vi "GetMicronArgs.vi"(8 "error in (no error)":errorcluster, 10 "Args":string[](array[string]), 11 "Default Connection String":string="localhost:50051") -> (0 "error out":errorcluster, 3 "Micron Args":T1)   [LabVIEW 2019, in "MicronServer.lvlib" / "ServiceBase.lvclass"]
uses:
  ServiceBase.lvclass
  Typedefs/MicronArgs.ctl
  <vilib>/Wiresmith Technology/G CLI/Argument Parser/Option Class/Option Configuration.ctl
  <vilib>/Wiresmith Technology/G CLI/Argument Parser/Option Class/Argument Type.ctl
  <vilib>/SLL Toolkit/SLL String/_SubVIs/String to 1D String Array.vi
  <vilib>/SLL Toolkit/SLL String/_SubVIs/String to I32.vi
  <vilib>/Wiresmith Technology/G CLI/Argument Parser/Option Set Class/Option Set.lvclass
  <vilib>/Wiresmith Technology/G CLI/Argument Parser/Option Class/Option.lvclass
  <vilib>/SLL Toolkit/SLL String/SLL String.lvlib
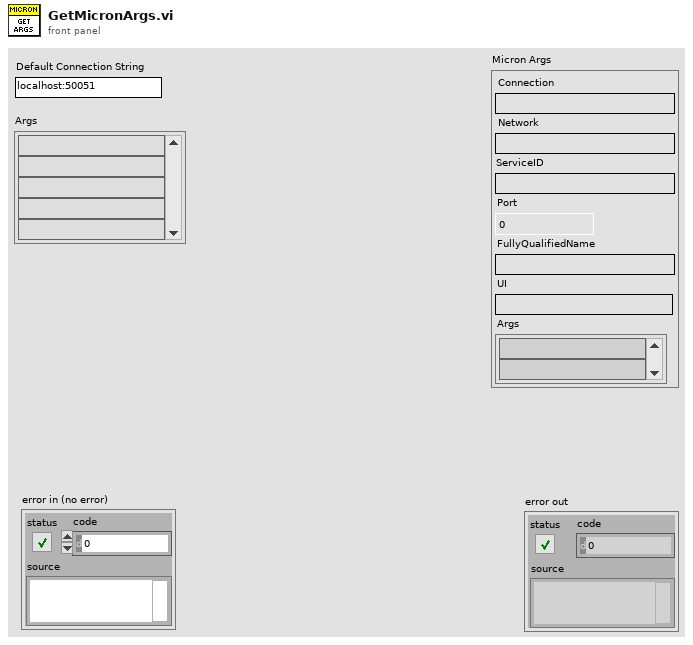
[diagram p1: front panel]
types:
  T1 = typedef "MicronServer.lvlib/ServiceBase.lvclass/MicronArgs.ctl" = cluster{"Connection":string, "Network":string, "ServiceID":string, "Port":i32, "FullyQualifiedName":string, "UI":string, "Args":string[]}
  T2 = typedef "Option Parser.lvlib/Option.lvclass/Argument Type.ctl" = enum16{"flag", "value"}
  T3 = typedef "Option Parser.lvlib/Option.lvclass/Option Configuration.ctl" = cluster{"Option Type":T2, "Option Labels":string[], "Key":string, "Description":string, "Required":bool, "Default Value":string}
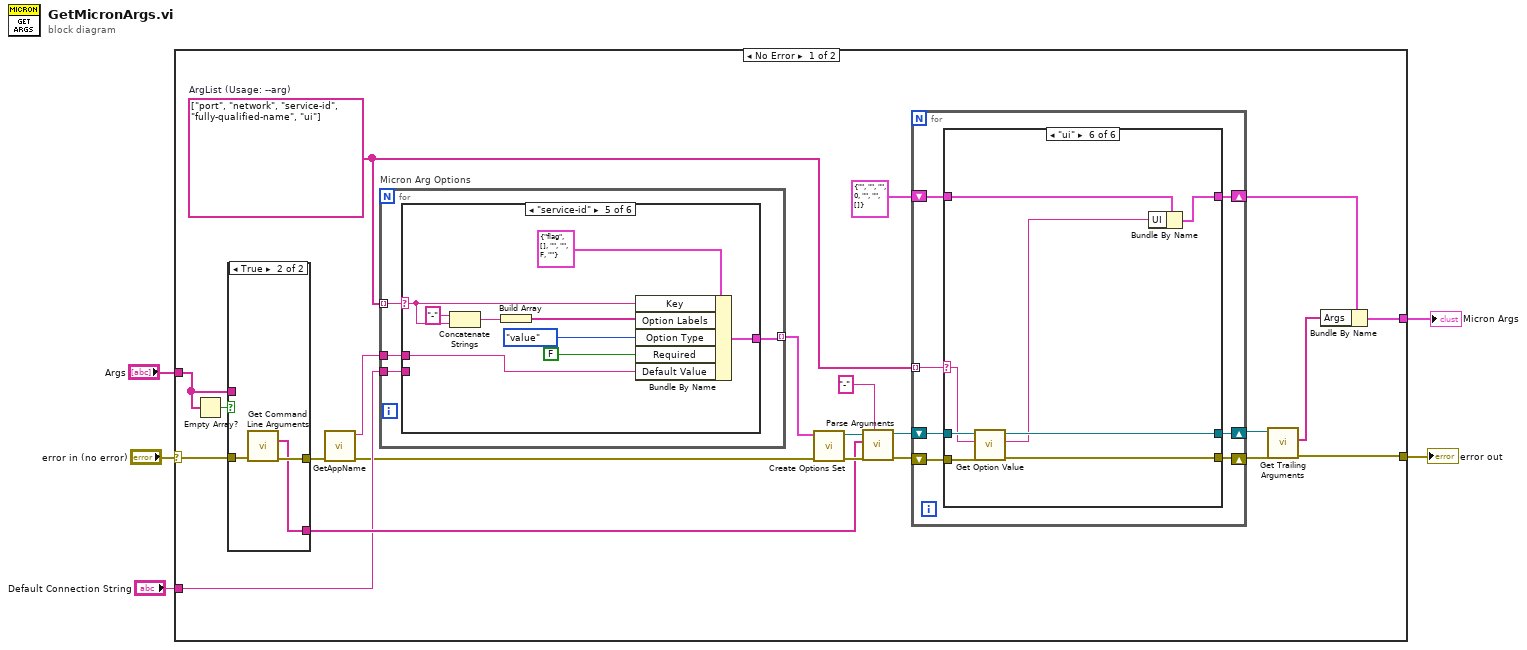
[diagram p0: block diagram]
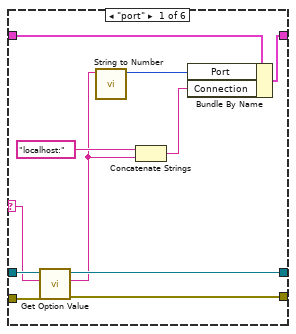
[diagram p3: hidden frame]
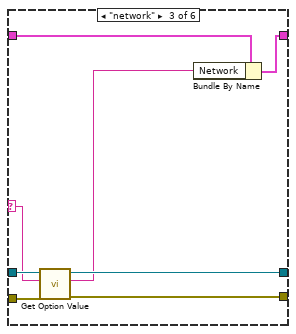
[diagram p5: hidden frame]
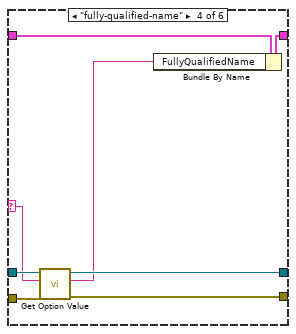
[diagram p6: hidden frame]
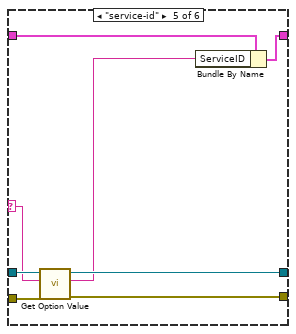
[diagram p7: hidden frame]
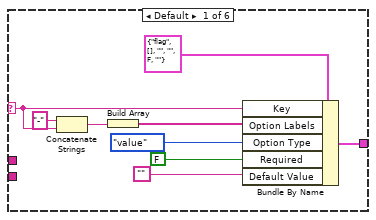
[diagram p8: hidden frame]
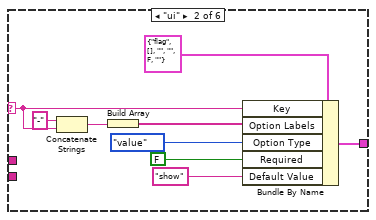
[diagram p9: hidden frame]
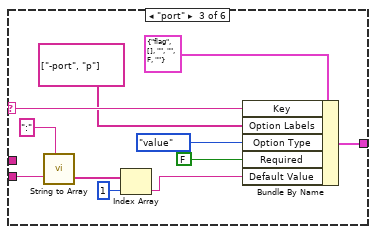
[diagram p10: hidden frame]
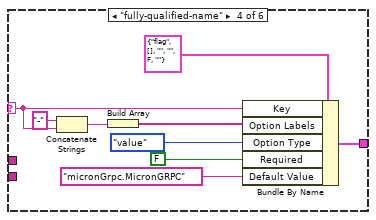
[diagram p11: hidden frame]
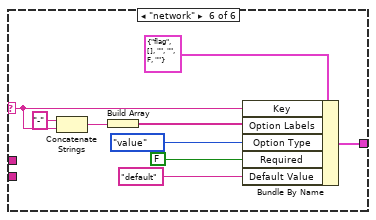
[diagram p12: hidden frame]
diagram:
  n1 = case shown="No Error" "error in (no error)" {
    selector: "error in (no error)" -> [w27 w146]
    tunnel: [w14 w146] -> w4
    tunnel: [w16 _] -> w3
    tunnel: "Args" -> [w10 _]
    tunnel: "Default Connection String" -> [w9 _]
    frame No Error {
      w21 = string[] ["port", "network", "service-id", "fully-qualified-name", "ui"]  # ArgList (Usage: --arg)
      n2 = Empty Array?(array=w10) -> (empty?=w11:bool)
      n3 = case shown="True" w11 {
        tunnel: w27 -> [w28 w32]
        tunnel: [w28 w31] -> w8
        tunnel: [w29 w30] -> w12
        tunnel: w10 -> [w29 _]
        frame False {
        }
        frame True {
          n4 = call <vilib>:"Get Command Line Arguments.vi"("error in (no error)"=w32) -> ("error out"=w31:errorcluster, "arguments"=w30:string[])  [unwired: 8 in, 1 out]
        }
      }
      n5 = call "GetAppName.vi"("error in (no error)"=w8) -> ("error out"=w7:errorcluster, "AppName"=w6:string)  [unwired: 9 in]
      n6 = for "Micron Arg Options" {
        tunnel: w21 -> [w89] mode=indexing
        tunnel: [w88] -> w22 mode=indexing
        tunnel: w9 -> [w87]
        tunnel: w6 -> [w86]
        n7 = case shown="\"service-id\"" w89 {
          selector: w89 -> [w91 w101 w114 w121 w130 w139]
          tunnel: [w97 w106 w117 w126 w135 w144] -> w88
          tunnel: w87 -> [_ _ w112 _ _ _]
          tunnel: w86 -> [_ _ _ _ w128 _]
          frame Default {
            n8 = Concatenate Strings("-" ("string"), w91) -> (w92:string)
            n9 = Build Array(w92) -> (w96:string[])
            n10 = Bundle By Name(cluster=T3 {"Option Type"=enum."flag", "Option Labels"=[], "Key"="", "Description"="", "Required"=FALSE, "Default Value"=""} ("Option Config"), "Key"=w91, "Option Labels"=w96, "Option Type"=Argument_Type."value", "Required"=FALSE, "Default Value"="") -> (w97:T3)
          }
          frame "ui" {
            n11 = Concatenate Strings("-" ("string"), w101) -> (w102:string)
            n12 = Build Array(w102) -> (w105:string[])
            n13 = Bundle By Name(cluster=T3 {"Option Type"=enum."flag", "Option Labels"=[], "Key"="", "Description"="", "Required"=FALSE, "Default Value"=""} ("Option Config"), "Key"=w101, "Option Labels"=w105, "Option Type"=Argument_Type."value", "Required"=FALSE, "Default Value"="show") -> (w106:T3)
          }
          frame "port" {
            n14 = call-poly <vilib>:"String to Array.vi"("Delimiter (,)"=":", "String"=w112) -> ("Array[]"=w110:string[])  [unwired: 6 in]
            n15 = Index Array(array=w110, index=1) -> (element=w108:string)
            n16 = Bundle By Name(cluster=T3 {"Option Type"=enum."flag", "Option Labels"=[], "Key"="", "Description"="", "Required"=FALSE, "Default Value"=""} ("Option Config"), "Key"=w114, "Option Labels"=string[] ["-port", "p"], "Option Type"=Argument_Type."value", "Required"=FALSE, "Default Value"=w108) -> (w117:T3)
          }
          frame "fully-qualified-name" {
            n17 = Concatenate Strings("-" ("string"), w121) -> (w122:string)
            n18 = Build Array(w122) -> (w125:string[])
            n19 = Bundle By Name(cluster=T3 {"Option Type"=enum."flag", "Option Labels"=[], "Key"="", "Description"="", "Required"=FALSE, "Default Value"=""} ("Option Config"), "Key"=w121, "Option Labels"=w125, "Option Type"=Argument_Type."value", "Required"=FALSE, "Default Value"="micronGrpc.MicronGRPC") -> (w126:T3)
          }
          frame "service-id" {
            n20 = Concatenate Strings("-" ("string"), w130) -> (w131:string)
            n21 = Build Array(w131) -> (w134:string[])
            n22 = Bundle By Name(cluster=T3 {"Option Type"=enum."flag", "Option Labels"=[], "Key"="", "Description"="", "Required"=FALSE, "Default Value"=""} ("Option Config"), "Key"=w130, "Option Labels"=w134, "Option Type"=Argument_Type."value", "Required"=FALSE, "Default Value"=w128) -> (w135:T3)
          }
          frame "network" {
            n23 = Concatenate Strings("-" ("string"), w139) -> (w140:string)
            n24 = Build Array(w140) -> (w143:string[])
            n25 = Bundle By Name(cluster=T3 {"Option Type"=enum."flag", "Option Labels"=[], "Key"="", "Description"="", "Required"=FALSE, "Default Value"=""} ("Option Config"), "Key"=w139, "Option Labels"=w143, "Option Type"=Argument_Type."value", "Required"=FALSE, "Default Value"="default") -> (w144:T3)
          }
        }
      }
      n26 = call <vilib>:"Create Options Set.vi"("error in (no error)"=w7, "Options"=w22) -> ("error out"=w26:errorcluster, "Option Set out"=w25:refnum<class "Option Set.lvclass">)  [unwired: 8 in]
      n27 = call <vilib>:"Parse Arguments.vi"("Label Marker (-)"="-", "error in (no error)"=w26, "Arguments"=w12, "Option Set in"=w25) -> ("error out"=w23:errorcluster, "Option Set out"=w24:refnum<class "Option Set.lvclass">)  [unwired: 4 in, 2 out]
      n28 = for {
        shift-right: [w37] -> w18
        shift-left: w24 -> [w39]
        shift-right: [w36] -> w19
        shift-left: w23 -> [w38]
        tunnel: w21 -> [w35] mode=indexing
        shift-right: [w33] -> w17
        shift-left: T1 {"Connection"="", "Network"="", "ServiceID"="", "Port"=0, "FullyQualifiedName"="", "UI"="", "Args"=[]} ("Micron Args") -> [w34]
        n29 = case shown="\"ui\"" w35 {
          selector: w35 -> [w46 _ w57 w65 w73 w81]
          tunnel: w39 -> [w50 w52 w61 w69 w77 w85]
          tunnel: w38 -> [w49 w51 w60 w68 w76 w84]
          tunnel: [w48 w52 w59 w67 w75 w83] -> w37
          tunnel: [w47 w51 w58 w66 w74 w82] -> w36
          tunnel: w34 -> [w45 w53 w56 w64 w72 w80]
          tunnel: [w44 w53 w55 w63 w71 w79] -> w33
          frame "port" {
            n30 = call <vilib>:"Get Option Value.vi"("error in (no error)"=w49, "Option Key"=w46, "Option Set in"=w50) -> ("error out"=w47:errorcluster, "Value"=w41:string, "Option Set out"=w48:refnum<class "Option Set.lvclass">)  [unwired: 5 in, 1 out]
            n31 = call-poly <vilib>:"String to Number.vi"("String"=w41) -> ("Numeric"=w43:i32)  [unwired: 10 in]
            n32 = Concatenate Strings("localhost:" ("string"), w41) -> (w40:string)
            n33 = Bundle By Name(cluster=w45, "Port"=w43, "Connection"=w40) -> (w44:T1)
          }
          frame Default {
          }
          frame "network" {
            n34 = call <vilib>:"Get Option Value.vi"("error in (no error)"=w60, "Option Key"=w57, "Option Set in"=w61) -> ("error out"=w58:errorcluster, "Value"=w54:string, "Option Set out"=w59:refnum<class "Option Set.lvclass">)  [unwired: 5 in, 1 out]
            n35 = Bundle By Name(cluster=w56, "Network"=w54) -> (w55:T1)
          }
          frame "fully-qualified-name" {
            n36 = call <vilib>:"Get Option Value.vi"("error in (no error)"=w68, "Option Key"=w65, "Option Set in"=w69) -> ("error out"=w66:errorcluster, "Value"=w62:string, "Option Set out"=w67:refnum<class "Option Set.lvclass">)  [unwired: 5 in, 1 out]
            n37 = Bundle By Name(cluster=w64, "FullyQualifiedName"=w62) -> (w63:T1)
          }
          frame "service-id" {
            n38 = call <vilib>:"Get Option Value.vi"("error in (no error)"=w76, "Option Key"=w73, "Option Set in"=w77) -> ("error out"=w74:errorcluster, "Value"=w70:string, "Option Set out"=w75:refnum<class "Option Set.lvclass">)  [unwired: 5 in, 1 out]
            n39 = Bundle By Name(cluster=w72, "ServiceID"=w70) -> (w71:T1)
          }
          frame "ui" {
            n40 = call <vilib>:"Get Option Value.vi"("error in (no error)"=w84, "Option Key"=w81, "Option Set in"=w85) -> ("error out"=w82:errorcluster, "Value"=w78:string, "Option Set out"=w83:refnum<class "Option Set.lvclass">)  [unwired: 5 in, 1 out]
            n41 = Bundle By Name(cluster=w80, "UI"=w78) -> (w79:T1)
          }
        }
      }
      n42 = call <vilib>:"Get Trailing Arguments.vi"("error in (no error)"=w19, "Option Set in"=w18) -> ("error out"=w14:errorcluster, "Arguments"=w15:string[])  [unwired: 7 in, 1 out]
      n43 = Bundle By Name(cluster=w17, "Args"=w15) -> (w16:T1)
    }
    frame Error {
    }
  }
  "error out" <- w4
  "Micron Args" <- w3
